vi "Save File Save Data.vi"(6 "New File Created":bool, 9 "Data":string[](array[string]), 10 "Header":string[](array[string]), 11 "Debug File Path":path) -> ()   [LabVIEW 2016]
uses:
  <vilib>/Utility/file.llb/Write To Spreadsheet File (string).vi
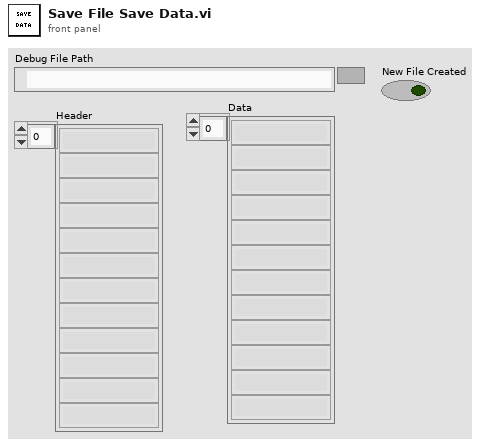
[diagram p1: front panel]
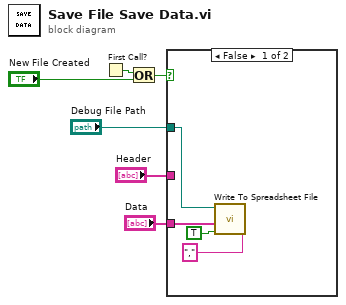
[diagram p0: block diagram]
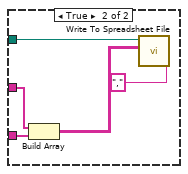
[diagram p2: hidden frame]
diagram:
  n1 = First Call?() -> (First Call?: T/F=w1:bool)
  n2 = Or(x=w1, y="New File Created") -> (x .or. y?=w3:bool)
  n3 = case shown="False" w3 {
    tunnel: "Data" -> [w9 w15]
    tunnel: "Debug File Path" -> [w10 w14]
    tunnel: "Header" -> [_ w12]
    frame False {
      n4 = call-poly <vilib>:"Write To Spreadsheet File.vi"("delimiter (\\t)"="," ("delimiter (\\t)"), "append to file? (new file:F)"=TRUE, "1D data"=w9, "file path (dialog if empty)"=w10) -> ()  [unwired: 4 in, 1 out]
    }
    frame True {
      n5 = Build Array(w12, w15) -> (w11:string[][])
      n6 = call-poly <vilib>:"Write To Spreadsheet File.vi"("delimiter (\\t)"="," ("delimiter (\\t)"), "2D data"=w11, "file path (dialog if empty)"=w14) -> ()  [unwired: 5 in, 1 out]
    }
  }
